vi "ValidateSignature.vi"(8 "error in (no error)":errorcluster, 9 "Signature to validate":string, 10 "Data to Validate":variant, 11 "CryptoType":refnum<class "Signature.lvclass">) -> (0 "error out":errorcluster, 2 "Valid Signature":bool)   [LabVIEW 2016, in "Signature.lvclass"]
uses:
  Signature.lvclass
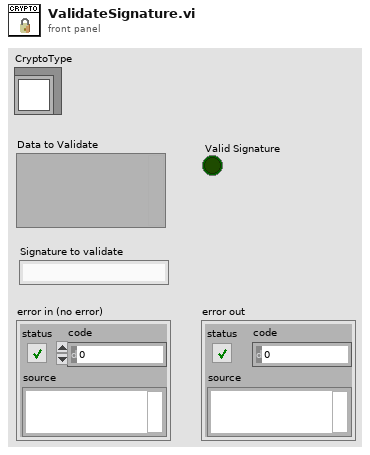
[diagram p1: front panel]
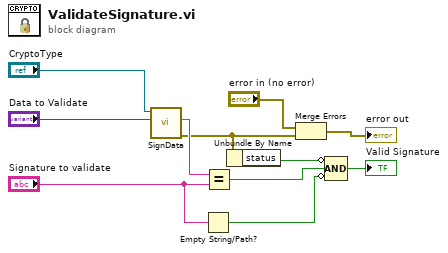
[diagram p0: block diagram]
diagram:
  n1 = call-dynamic "SignData.vi"("Data to Sign"="Data to Validate", "CryptoType"="CryptoType") -> ("error out"=w4:errorcluster, "Signature"=w9:string)  [unwired: 8 in]
  n2 = Empty String/Path?(string/path="Signature to validate") -> (empty?=w6:bool)
  n3 = Equal?(x=w9, y="Signature to validate") -> (x = y?=w8:bool)
  n4 = Unbundle By Name(w4) -> ("status"=w3:bool)
  n5 = Merge Errors("error in (no error)", w4) -> (→"error out":errorcluster)
  n6 = Compound Arithmetic op=AND(invert w3, w8, invert w6) -> (→"Valid Signature":bool)
